vi "RegStateEvent.vi"(8 "error in":errorcluster, 10 "StateEvent":T1, 11 "States":T2) -> (0 "error out":errorcluster, 2 "StateEvent(out)":T1, 3 "Event Registration Refnum":refnum<event-registration>)   [LabVIEW 2009]
uses:
  Controls/States.ctl
  Controls/StateEvents.ctl
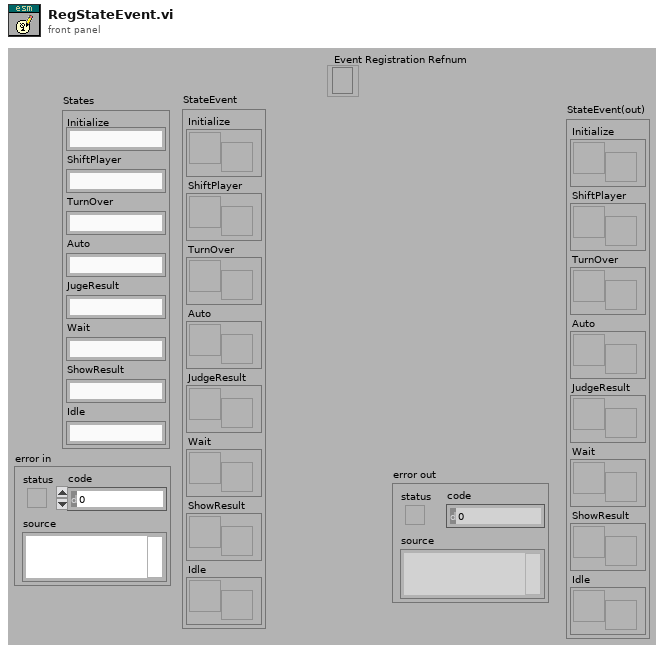
[diagram p1: front panel]
types:
  T1 = typedef "StateEvents.ctl" = cluster{"Initialize":refnum<user-event>, "ShiftPlayer":refnum<user-event>, "TurnOver":refnum<user-event>, "Auto":refnum<user-event>, "JudgeResult":refnum<user-event>, "Wait":refnum<user-event>, "ShowResult":refnum<user-event>, "Idle":refnum<user-event>}
  T2 = typedef "States.ctl" = cluster{"Initialize":string, "ShiftPlayer":string, "TurnOver":string, "Auto":string, "JugeResult":string, "Wait":string, "ShowResult":string, "Idle":string}
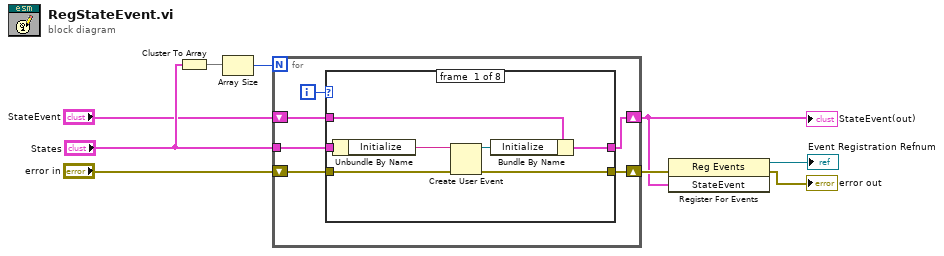
[diagram p0: block diagram]
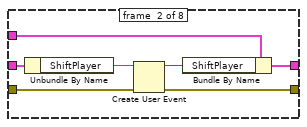
[diagram p2: hidden frame]
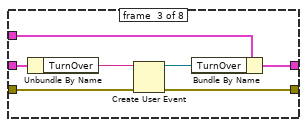
[diagram p3: hidden frame]
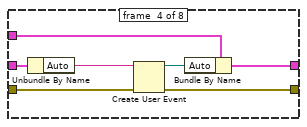
[diagram p4: hidden frame]
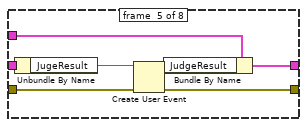
[diagram p5: hidden frame]
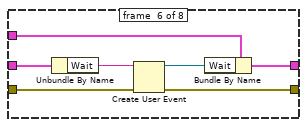
[diagram p6: hidden frame]
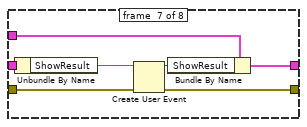
[diagram p7: hidden frame]
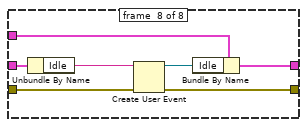
[diagram p8: hidden frame]
diagram:
  n1 = Cluster To Array(cluster="States") -> (array=w9:string[])
  n2 = Array Size(array=w9) -> (size(s)=w8:i32)
  n3 = for {
    N: w8 -> [_]
    tunnel: "States" -> [w14]
    shift-right: [w12] -> w2
    shift-left: "StateEvent" -> [w13]
    shift-right: [w10] -> w4
    shift-left: "error in" -> [w11]
    i -> [w15]
    n4 = case shown="7" w15 {
      tunnel: w14 -> [w19 w28 w33 w40 w47 w54 w61 w68]
      tunnel: w13 -> [w20 w29 w34 w41 w48 w55 w62 w69]
      tunnel: [w18 w27 w32 w39 w46 w53 w60 w67] -> w12
      tunnel: w11 -> [w17 w24 w31 w38 w45 w52 w59 w66]
      tunnel: [w16 w23 w30 w37 w44 w51 w58 w65] -> w10
      frame #0 {
        n5 = Unbundle By Name(w19) -> ("Initialize"=w21:string)
        n6 = Create User Event(user event datatype=w21, error in=w17) -> (user event=w22:refnum<user-event>, error out=w16:errorcluster)
        n7 = Bundle By Name(cluster=w20, "Initialize"=w22) -> (w18:T1)
      }
      frame #1 {
        n8 = Unbundle By Name(w28) -> ("ShiftPlayer"=w26:string)
        n9 = Create User Event(user event datatype=w26, error in=w24) -> (user event=w25:refnum<user-event>, error out=w23:errorcluster)
        n10 = Bundle By Name(cluster=w29, "ShiftPlayer"=w25) -> (w27:T1)
      }
      frame #2 {
        n11 = Unbundle By Name(w33) -> ("TurnOver"=w35:string)
        n12 = Create User Event(user event datatype=w35, error in=w31) -> (user event=w36:refnum<user-event>, error out=w30:errorcluster)
        n13 = Bundle By Name(cluster=w34, "TurnOver"=w36) -> (w32:T1)
      }
      frame #3 {
        n14 = Unbundle By Name(w40) -> ("Auto"=w42:string)
        n15 = Create User Event(user event datatype=w42, error in=w38) -> (user event=w43:refnum<user-event>, error out=w37:errorcluster)
        n16 = Bundle By Name(cluster=w41, "Auto"=w43) -> (w39:T1)
      }
      frame #4 {
        n17 = Unbundle By Name(w47) -> ("JugeResult"=w49:string)
        n18 = Create User Event(user event datatype=w49, error in=w45) -> (user event=w50:refnum<user-event>, error out=w44:errorcluster)
        n19 = Bundle By Name(cluster=w48, "JudgeResult"=w50) -> (w46:T1)
      }
      frame #5 {
        n20 = Unbundle By Name(w54) -> ("Wait"=w56:string)
        n21 = Create User Event(user event datatype=w56, error in=w52) -> (user event=w57:refnum<user-event>, error out=w51:errorcluster)
        n22 = Bundle By Name(cluster=w55, "Wait"=w57) -> (w53:T1)
      }
      frame #6 {
        n23 = Unbundle By Name(w61) -> ("ShowResult"=w63:string)
        n24 = Create User Event(user event datatype=w63, error in=w59) -> (user event=w64:refnum<user-event>, error out=w58:errorcluster)
        n25 = Bundle By Name(cluster=w62, "ShowResult"=w64) -> (w60:T1)
      }
      frame #7 {
        n26 = Unbundle By Name(w68) -> ("Idle"=w70:string)
        n27 = Create User Event(user event datatype=w70, error in=w66) -> (user event=w71:refnum<user-event>, error out=w65:errorcluster)
        n28 = Bundle By Name(cluster=w69, "Idle"=w71) -> (w67:T1)
      }
    }
  }
  "StateEvent(out)" <- w2
  n29 = register-events(error in=w4, w2) -> (reference out=→"Event Registration Refnum":refnum<event-registration>, error out=→"error out":errorcluster)  [unwired: 1 in]
